vi "Write to USB Cards.vi"(0 "physical channels":refnum<k21>="Dev0/Ao0:15", 1 "physical channels 2":refnum<k21>="Dev1/Ao0:15", 2 "Array":dbl[](array[numeric])=[0.0, 0.0, 0.0, 0.0, 0.0, 0.0, 0.0, 0.0, 0.0, 0.0, 0.0, 0.0, 0.0, 0.0, 0.0, 0.0, 0.0, 0.0, 0.0, 0.0, 0.0, 0.0, 0.0, 0.0, 0.0, 0.0, 0.0, 0.0, 0.0, 0.0, 0.0, 0.0], 3 "error in":errorcluster) -> (9 "error out":errorcluster={"status"=TRUE, "code"=100000, "source"="ULx Stop Task.vi<ERR>\nMeasurements: Value passed to the Task I/O In control is an empty I/O task).\n\nThe value must refer to a valid task."})   [LabVIEW 2016]
uses:
  <vilib>/ULx/Create Channel.llb/ULx Create Channel (AO-Voltage-Basic).vi
  <vilib>/ULx/Write.llb/ULx Write (Analog 1D DBL NChan 1Samp).vi
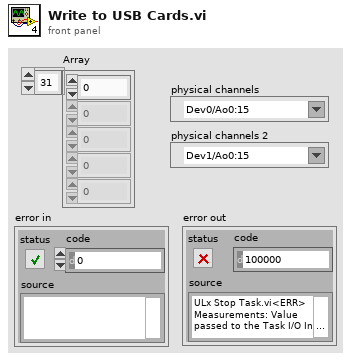
[diagram p1: front panel]
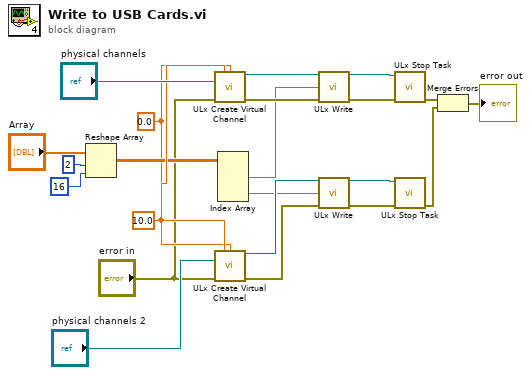
[diagram p0: block diagram]
diagram:
  w3 = 0.0 ("minimum value")
  w21 = 10.0 ("maximum value")
  n1 = Reshape Array("Array", 2 ("dimension size"), 16 ("dimension size")) -> (w13:dbl[][])
  n2 = call-poly <vilib>:"ULx Create Virtual Channel.vi"("maximum value"=w21, "minimum value"=w3, "physical channels"="physical channels", "error in"="error in") -> ("task out"=w1:refnum<k24>, "error out"=w17:errorcluster)  [unwired: 10 in]
  n3 = call-poly <vilib>:"ULx Create Virtual Channel.vi"("maximum value"=w21, "minimum value"=w3, "physical channels"="physical channels 2", "error in"="error in") -> ("task out"=w19:refnum<k24>, "error out"=w18:errorcluster)  [unwired: 10 in]
  n4 = Index Array(array=w13) -> (element #1=w12:dbl[], element #2=w11:dbl[])  [unwired: 4 in]
  n5 = call-poly <vilib>:"ULx Write.vi"("task in"=w1, "data"=w12, "error in"=w17) -> ("task out"=w10:refnum<k24>, "error out"=w9:errorcluster)  [unwired: 10 in, 1 out]
  n6 = call-poly <vilib>:"ULx Write.vi"("task in"=w19, "data"=w11, "error in"=w18) -> ("task out"=w8:refnum<k24>, "error out"=w7:errorcluster)  [unwired: 10 in, 1 out]
  n7 = call <vilib>:"ULx Stop Task.vi"("error in"=w9, "task in"=w10) -> ("error out"=w6:errorcluster)  [unwired: 8 in, 1 out]
  n8 = call <vilib>:"ULx Stop Task.vi"("error in"=w7, "task in"=w8) -> ("error out"=w5:errorcluster)  [unwired: 8 in, 1 out]
  n9 = Merge Errors(w6, w5) -> (→"error out":errorcluster)
